vi "Lockin diagnosis.vi"() -> ()   [LabVIEW 2010]
panel:
  in  "Write to file?":bool
  in  "Loop Delay":dbl
  in  "Configure lockin":T1(tab)
  out "range":string
  in  "Auto Sensitivity":bool
  in  "Update":bool
  in  "Auto Measure":bool
  out "Auto Sensitivity out":bool
  out "Auto Measure out":bool
  in  "Input Mode 2":i32(ring) items=["Voltage Input ( A or A-B)", "Current Input 10E6 V/A", "Current Input 10E8 V/A"]
  in  "Range 2":i32(ring)=13 items=["100 nV", "300 nV", "1 uV", "3 uV", "10 uV", "30 uV", "100 uV", "300 uV", "1 mV", "3 mV", "10 mV", "30 mV", "100 mV", "300 mV", "1 V", "3 V"]
  in  "Ring":u16(ring) items=["OFF", "2F", "F", "F & 2F"]
  in  "Update?":bool
  in  "ON":bool
  in  "Update?":bool
  in  "Range":i32(ring)=13 items=["100 nV", "300 nV", "1 uV", "3 uV", "10 uV", "30 uV", "100 uV", "300 uV", "1 mV", "3 mV", "10 mV", "30 mV", "100 mV", "300 mV", "1 V", "3 V"]
  in  "display type":i32(ring)=1 items=["Output %", "Output calibrated ", "Ratio", "log Ratio", "ADC 1", "ADC 2", " ADC 3", "ADC 4", "Noise %", "Noise Calibrated", "Ref. Frequency"]
  in  "time constant":i32(ring) items=["1 ms", "3 ms", "10 ms", "30 ms", "100 ms", "300 ms", "1 s", "3 s", "10 s", "30 s", "100 s", "300 s", "1 ks", "3 ks"]
  in  "Input Mode":i32(ring) items=["Voltage Input ( A or A-B)", "Current Input 10E6 V/A", "Current Input 10E8 V/A"]
  in  "slope":i32(ring)=1 items=["6dB/octave", "12dB/octave"]
  out "Units":string
  out "Display":dbl
  out "Available Display Types Out":string[](array[string])
  out "VISA session":refnum<visa-resource-name>
  out "Display Precision":dbl
  out "error out":errorcluster
  out "Refereance unlock":bool
  out "Overload":bool
  out "Output":ext
  in  "Read?":bool
  in  "Initialize":bool
  in  "stop?":bool
  in  "GPIB Address Lock-In":u8=12 min=1 max=32 step=1
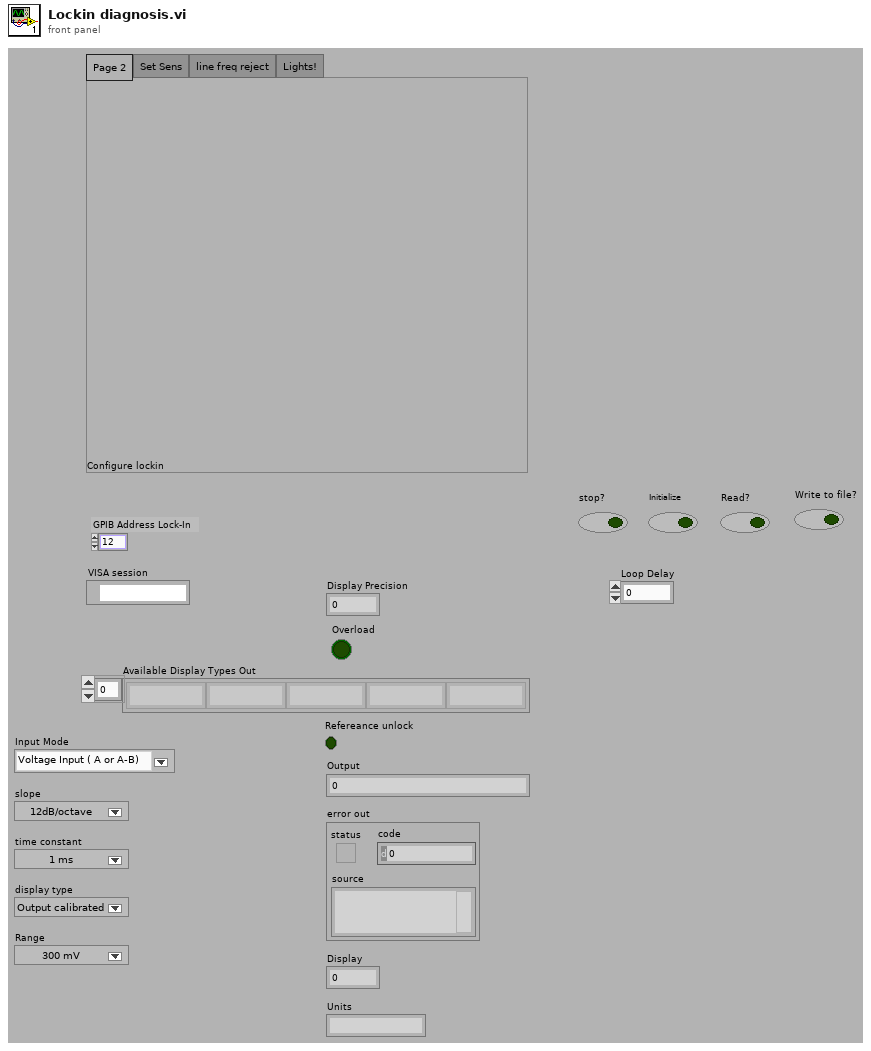
[diagram p1: front panel]
types:
  T1 = enum32{"Page 2", "Set Sens", "line freq reject", "Lights!"}
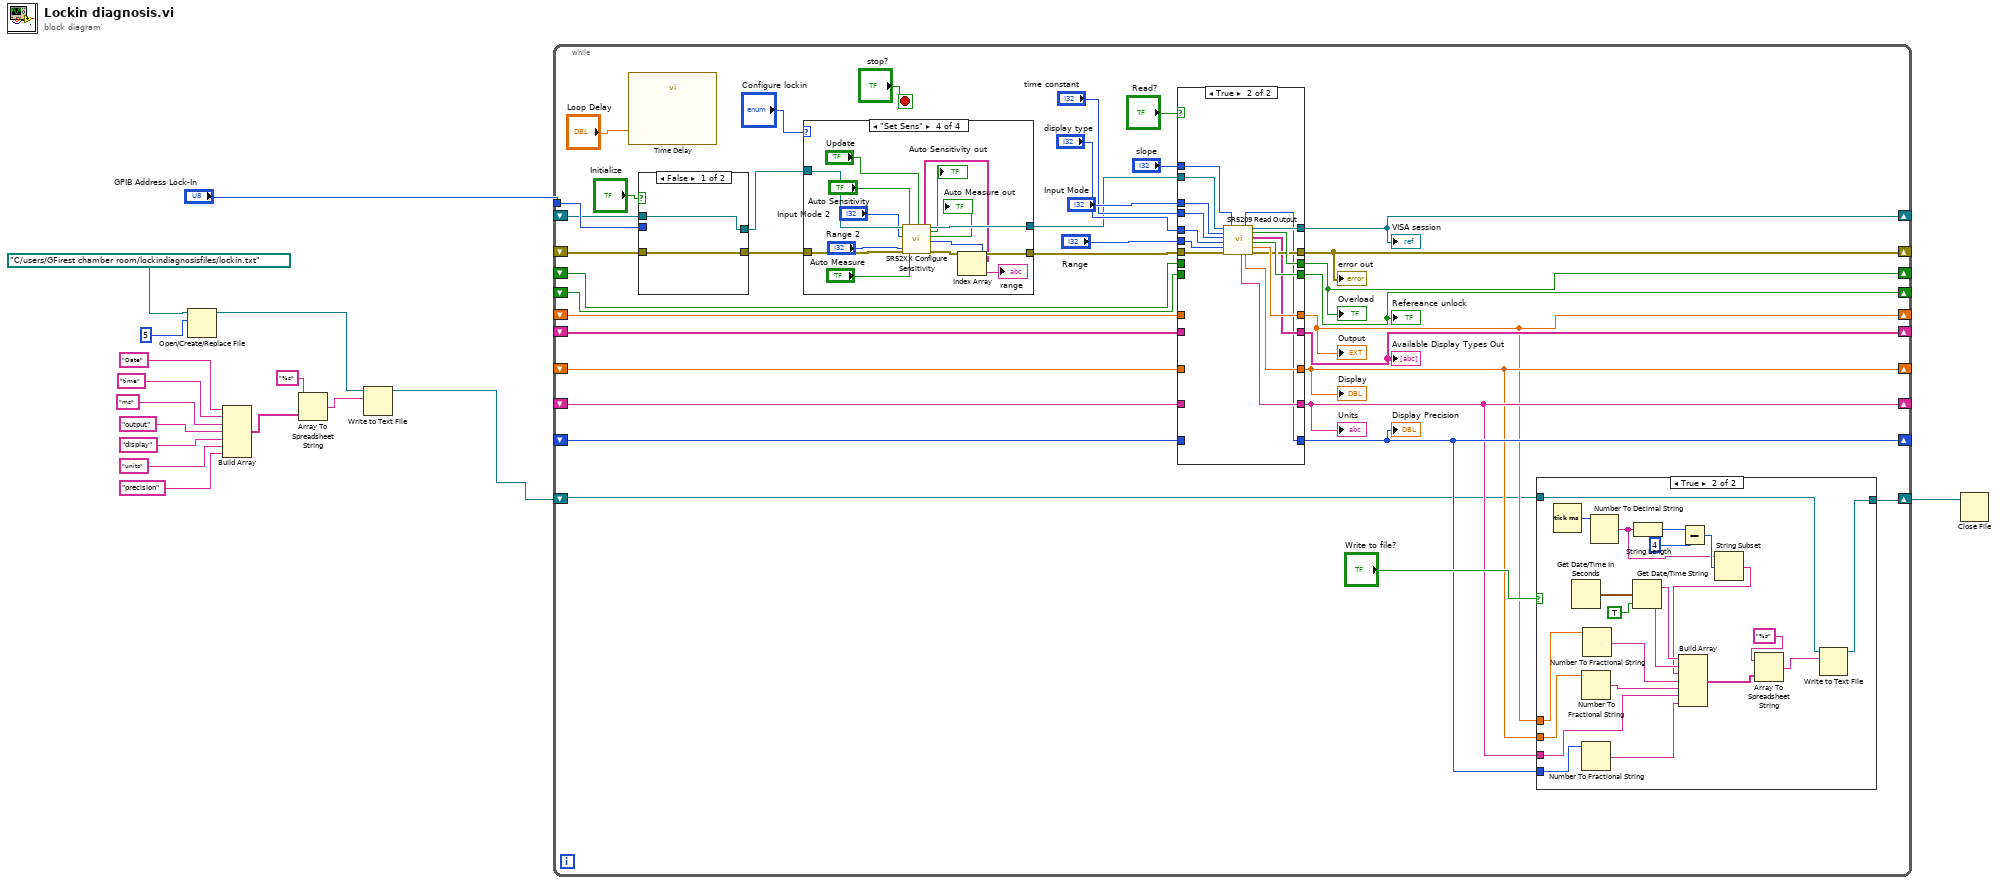
[diagram p0: block diagram]
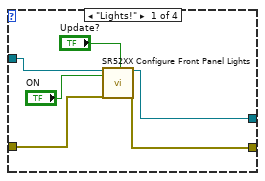
[diagram p3: hidden frame]
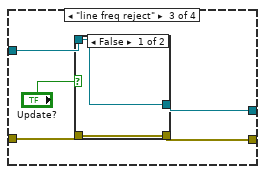
[diagram p5: hidden frame]
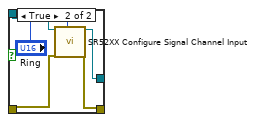
[diagram p6: hidden frame]
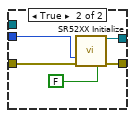
[diagram p8: hidden frame]
diagram:
  n1 = Open/Create/Replace File(file path (use dialog)=path "C:/users/GFirest chamber room/lockindiagnosisfiles/lockin.txt", operation (0:open)=5) -> (refnum out=w11:refnum<file>)  [unwired: 4 in, 2 out]
  n2 = Build Array("Date", "time", "ms", "output", "display", "units", "precision") -> (w9:string[])
  n3 = Array To Spreadsheet String(array=w9, 3:"%s") -> (spreadsheet string=w12:string)  [unwired: 1 in]
  n4 = Write to Text File(file (use dialog)=w11, text=w12) -> (refnum out=w10:refnum<file>)  [unwired: 2 in, 2 out]
  n5 = while {
    tunnel: "GPIB Address Lock-In" -> [w50]
    shift-right: [w48] -> _
    shift-left: _ -> [w42]
    shift-right: [w41] -> _
    shift-left: _ -> [w46]
    shift-right: [w19] -> _
    shift-left: _ -> [w43]
    shift-right: [w47] -> _
    shift-left: _ -> [w44]
    shift-right: [w36] -> _
    shift-left: _ -> [w45]
    shift-right: [w40] -> _
    shift-left: _ -> [w39]
    shift-right: [w20] -> _
    shift-left: _ -> [w38]
    shift-right: [w21] -> _
    shift-left: _ -> [w37]
    shift-right: [w22] -> _
    shift-left: _ -> [w35]
    shift-right: [w18] -> w14
    shift-left: w10 -> [w17]
    stop <- "stop?" stop-if-true
    n6 = call "Time Delay"("Delay Time (s)"="Loop Delay") -> ()  [unwired: 10 in, 1 out]
    n7 = case shown="False" "Initialize" {
      tunnel: w50 -> [_ w141]
      tunnel: [w136 w139] -> w28
      tunnel: w46 -> [w136 _]
      tunnel: w42 -> [w135 w138]
      tunnel: [w135 w137] -> w27
      frame False {
      }
      frame True {
        n8 = call "SR52XX Initialize"("Port"=w141, "error in (no error)"=w138, "reset"=FALSE) -> ("VISA session"=w139:refnum<visa-resource-name>, "error out"=w137:errorcluster)  [unwired: 10 in, 1 out]
      }
    }
    n9 = case shown="\"Set Sens\"" "Configure lockin" {
      tunnel: w28 -> [w79 w83 w88 w109]
      tunnel: w27 -> [w81 w82 w86 w108]
      tunnel: [w78 w83 w87 w106] -> w26
      tunnel: [w77 w82 w85 w107] -> w25
      frame "Lights!" {
        n10 = call "SR52XX Configure Front Panel Lights"("VISA session (for class)"=w79, "Lights"="ON", "error in (no error)"=w81, "Update"="Update?") -> ("dup VISA session"=w78:refnum<visa-resource-name>, "error out"=w77:errorcluster)  [unwired: 14 in]
      }
      frame "Page 2", Default {
      }
      frame "line freq reject" {
        n11 = case shown="False" "Update?" {
          tunnel: w88 -> [w89 w95]
          tunnel: [w89 w94] -> w87
          tunnel: w86 -> [w90 w93]
          tunnel: [w90 w92] -> w85
          frame False {
          }
          frame True {
            n12 = call "SR52XX Configure Signal Channel Input"("VISA session (for class)"=w95, "error in (no error)"=w93, "Line Frequency Rejection Filter"="Ring") -> ("VISA session"=w94:refnum<visa-resource-name>, "error out"=w92:errorcluster)  [unwired: 15 in]
          }
        }
      }
      frame "Set Sens" {
        n13 = call "SR52XX Configure Sensitivity"("VISA session (for class)"=w109, "Input Mode"="Input Mode 2", "Range"="Range 2", "error in (no error)"=w108, "Auto Sensitivity"="Auto Sensitivity", "Auto Measure"="Auto Measure", "Update"="Update") -> ("Range Annotations Out[]"=w98:string[], "VISA session"=w106:refnum<visa-resource-name>, "Auto Sensitivity out"=→"Auto Sensitivity out":bool, "Auto Measure out"=→"Auto Measure out":bool, "Range Out"=w97:u8, "error out"=w107:errorcluster)  [unwired: 7 in]
        n14 = Index Array(array=w98, index=w97) -> (element=→"range":string)
      }
    }
    n15 = case shown="True" "Read?" {
      tunnel: w26 -> [w114 w134]
      tunnel: [w116 w133] -> w19
      tunnel: [w117 w132] -> w47
      tunnel: [w118 w131] -> w36
      tunnel: [w115 w130] -> w48
      tunnel: w45 -> [w118 _]
      tunnel: w44 -> [w117 _]
      tunnel: w43 -> [w116 _]
      tunnel: w25 -> [w115 w129]
      tunnel: [w114 w128] -> w41
      tunnel: [w113 w127] -> w40
      tunnel: w39 -> [w113 _]
      tunnel: [w112 w126] -> w20
      tunnel: w38 -> [w112 _]
      tunnel: [w111 w125] -> w21
      tunnel: w37 -> [w111 _]
      tunnel: [w110 w124] -> w22
      tunnel: w35 -> [w110 _]
      tunnel: "slope" -> [_ w123]
      tunnel: "Input Mode" -> [_ w122]
      tunnel: "time constant" -> [_ w121]
      tunnel: "Range" -> [_ w120]
      tunnel: "display type" -> [_ w119]
      frame False {
      }
      frame True {
        n16 = call "SR5209 Read Output"("VISA session (for class)"=w134, "Input Mode"=w122, "Time Constant"=w121, "Display Type"=w119, "Range"=w120, "error in (no error)"=w129, "Slope"=w123) -> ("Units"=w125:string, "Display Precision"=w124:i32, "Display"=w126:dbl, "VISA session"=w128:refnum<visa-resource-name>, "Reference Unlock"=w131:bool, "Available Display Types Out"=w127:string[], "Overload"=w132:bool, "Output (FP)"=w133:dbl, "error out"=w130:errorcluster)  [unwired: 4 in]
      }
    }
    "Output" <- w19
    "Overload" <- w36
    "Refereance unlock" <- w47
    "error out" <- w48
    "Display Precision" <- w22
    "VISA session" <- w41
    "Available Display Types Out" <- w40
    "Display" <- w20
    "Units" <- w21
    n17 = case shown="True" "Write to file?" {
      tunnel: w22 -> [_ w73]
      tunnel: w21 -> [_ w68]
      tunnel: w20 -> [_ w74]
      tunnel: w19 -> [_ w75]
      tunnel: w17 -> [w53 w65]
      tunnel: [w53 w64] -> w18
      frame False {
      }
      frame True {
        n18 = Tick Count (ms)() -> (millisecond timer value=w57:u32)
        n19 = Get Date/Time In Seconds() -> (seconds since 1Jan1904=w63:timestamp)
        n20 = Number To Fractional String(number=w74) -> (F-format string=w69:string)  [unwired: 3 in]
        n21 = Number To Fractional String(number=w73) -> (F-format string=w67:string)  [unwired: 3 in]
        n22 = Number To Fractional String(number=w75) -> (F-format string=w70:string)  [unwired: 3 in]
        n23 = Number To Decimal String(number=w57) -> (decimal integer string=w55:string)  [unwired: 1 in]
        n24 = Get Date/Time String(seconds (now)=w63, want seconds? (F)=TRUE) -> (date string=w61:string, time string=w60:string)  [unwired: 1 in]
        n25 = String Length(string=w55) -> (length=w59:i32)
        n26 = Subtract(x=w59, y=4) -> (x-y=w56:i32)
        n27 = String Subset(string=w55, offset (0)=w56) -> (substring=w54:string)  [unwired: 1 in]
        n28 = Build Array(w61, w60, w54, w70, w69, w68, w67) -> (w72:string[])
        n29 = Array To Spreadsheet String(array=w72, 3:"%s") -> (spreadsheet string=w66:string)  [unwired: 1 in]
        n30 = Write to Text File(file (use dialog)=w65, text=w66) -> (refnum out=w64:refnum<file>)  [unwired: 2 in, 2 out]
      }
    }
  }
  n31 = Close File(refnum=w14) -> ()  [unwired: 1 in, 2 out]
